vi "Configure Measurement (Channel Power).vi"(0 "VISA resource name":refnum<visa-resource-name>, 5 "Channel Integration Bandwidth (2 MHz)":dbl=2000000.0 format="%#.6g", 7 "Channel Power Span (3 MHz)":dbl=3000000.0 format="%#.6g", 11 "error in (no error)":errorcluster) -> (4 "VISA resource name out":refnum<visa-resource-name>, 15 "error out":errorcluster)   [LabVIEW 2014, in "Agilent ESA PSA Series.lvlib"]
doc: "Sets up the channel power measurement operation."
uses:
  Agilent ESA PSA Series.lvlib
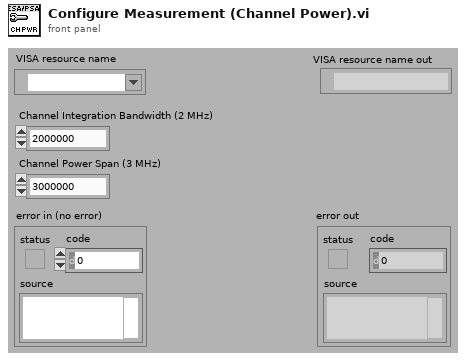
[diagram p1: front panel]
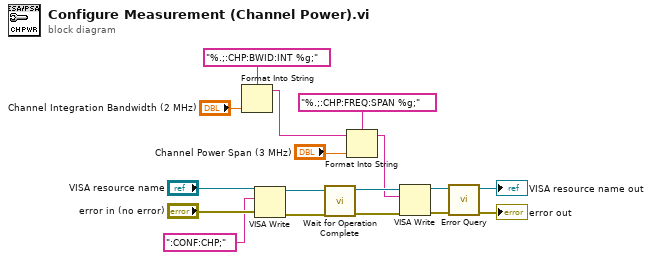
[diagram p0: block diagram]
diagram:
  n1 = Format Into String(format string="%.;:CHP:BWID:INT %g;", "Channel Integration Bandwidth (2 MHz)") -> (resulting string=w1:string)  [unwired: 2 in, 1 out]
  n2 = VISA Write(VISA resource name="VISA resource name", write buffer=":CONF:CHP;" ("initial string"), error in (no error)="error in (no error)") -> (VISA resource name out=w4:refnum<visa-resource-name>, error out=w5:errorcluster)  [unwired: 1 out]
  n3 = call "Wait for Operation Complete.vi"("error in (no error)"=w5, "VISA resource name"=w4) -> ("error out"=w9:errorcluster, "VISA resource name out"=w8:refnum<visa-resource-name>)  [unwired: 8 in]
  n4 = Format Into String(format string="%.;:CHP:FREQ:SPAN %g;", initial string=w1, "Channel Power Span (3 MHz)") -> (resulting string=w2:string)  [unwired: 1 in, 1 out]
  n5 = VISA Write(VISA resource name=w8, write buffer=w2, error in (no error)=w9) -> (VISA resource name out=w11:refnum<visa-resource-name>, error out=w10:errorcluster)  [unwired: 1 out]
  n6 = call "Error Query.vi"("error in (no error)"=w10, "VISA resource name"=w11) -> ("error out"=→"error out":errorcluster, "VISA resource name out"=→"VISA resource name out":refnum<visa-resource-name>)  [unwired: 6 in, 2 out]
